vi "Read config.vi"(8 "error in (no error)":errorcluster, 11 "FTPConfig in":refnum<class "FTPConfig.lvclass">) -> (0 "error out":errorcluster, 2 "FTP":T1={"address"="", "remote port"=21, "userName"="", "passWord"="", "RootDir"=""}, 3 "FTPConfig out":refnum<class "FTPConfig.lvclass">)   [LabVIEW 2020, in "FileSync -- FTP.lvlib" / "FTPConfig.lvclass"]
uses:
  FTPConfig.lvclass
  Def-FTP Server Info.vi
  FTPConfig.lvclass/FTPConfig.ctl
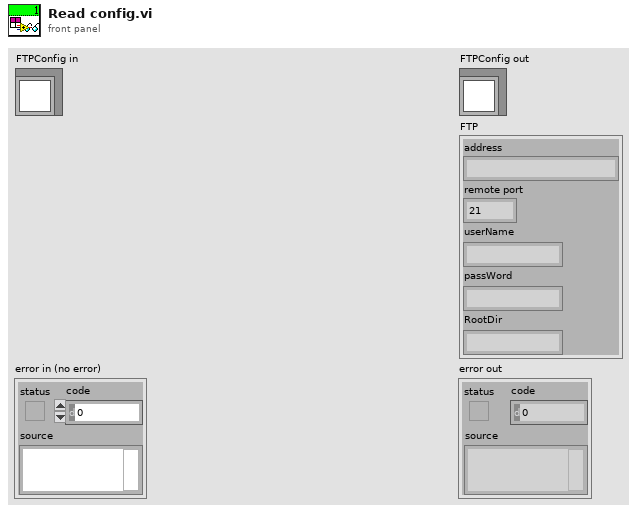
[diagram p1: front panel]
types:
  T1 = typedef "FileSync -- FTP.lvlib/FTPConfig.lvclass/Def-FTP Server Info.vi" = cluster{"address":string, "remote port":u16, "userName":string, "passWord":string, "RootDir":string}
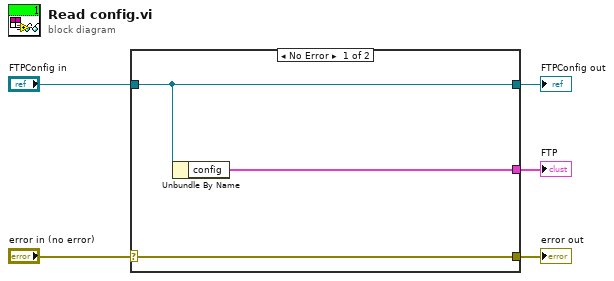
[diagram p0: block diagram]
diagram:
  n1 = case shown="No Error" "error in (no error)" {
    selector: "error in (no error)" -> [w8 w9]
    tunnel: [w8 w9] -> w4
    tunnel: [w7 w10] -> w2
    tunnel: "FTPConfig in" -> [w7 w10]
    tunnel: [w6 _] -> w1
    frame No Error {
      n2 = Unbundle By Name(w7) -> ("config"=w6:T1)
    }
    frame Error {
    }
  }
  "error out" <- w4
  "FTPConfig out" <- w2
  "FTP" <- w1
